vi "Read SensorID.vi"(8 "error in":errorcluster, 11 "cRIO repo in":refnum<class "cRIORepo.lvclass">) -> (0 "error out":errorcluster, 2 "sensor ID":string, 3 "cRIO repo out":refnum<class "cRIORepo.lvclass">)   [LabVIEW 2015, in "cRIORepo.lvclass"]
uses:
  cRIORepo.lvclass
  cRIORepo.lvclass/cRIORepo.ctl
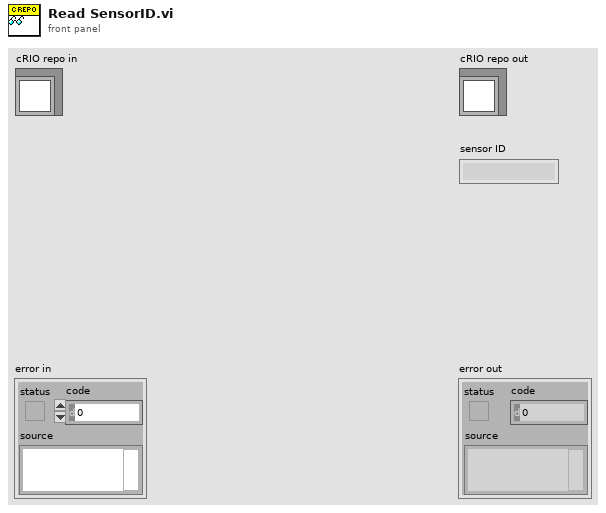
[diagram p1: front panel]
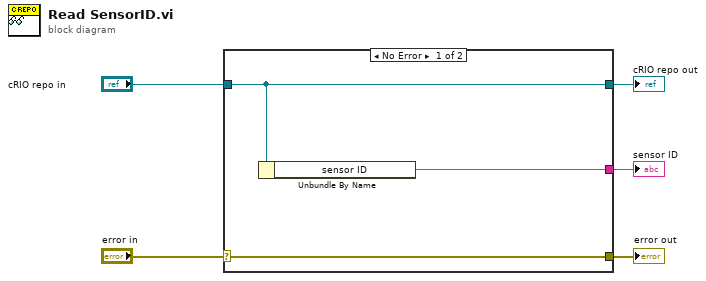
[diagram p0: block diagram]
diagram:
  n1 = case shown="No Error" "error in" {
    selector: "error in" -> [w8 w9]
    tunnel: [w8 w9] -> w4
    tunnel: [w7 w10] -> w2
    tunnel: "cRIO repo in" -> [w7 w10]
    tunnel: [w6 _] -> w1
    frame No Error {
      n2 = Unbundle By Name(w7) -> ("sensor ID"=w6:string)
    }
    frame Error {
    }
  }
  "error out" <- w4
  "cRIO repo out" <- w2
  "sensor ID" <- w1
